vi "Remove JSON Tag.vi"(11 "Name":string) -> (2 "Tag":T1, 3 "Name (tag stripped)":string)   [LabVIEW 2024, in "JSONtext.lvlib"]
uses:
  JSONtext.lvlib
  Tag Type.ctl
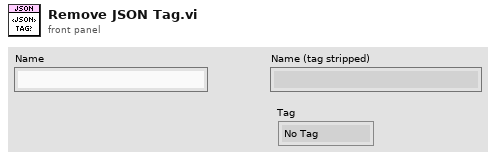
[diagram p1: front panel]
types:
  T1 = typedef "JSONtext.lvlib/Tag Type.ctl" = enum16{"No Tag", "<JSON>", "<JOBJ>", "<UTF8>"}
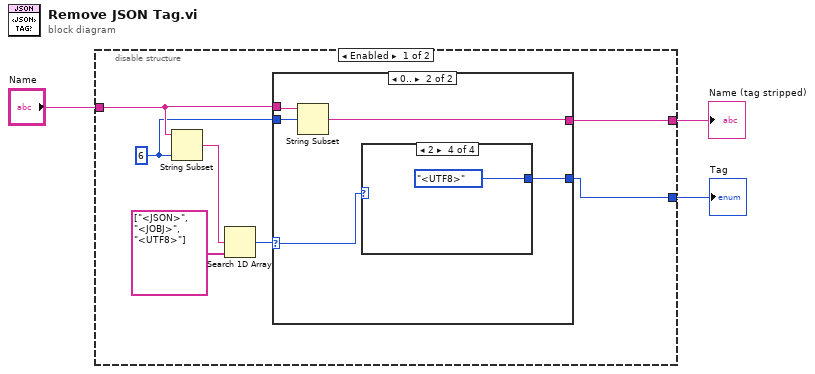
[diagram p0: block diagram]
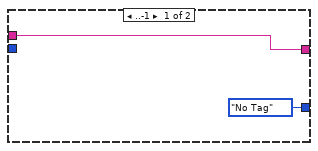
[diagram p2: hidden frame]
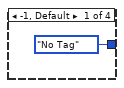
[diagram p3: hidden frame]
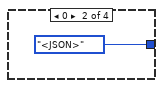
[diagram p4: hidden frame]
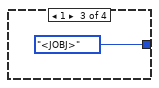
[diagram p5: hidden frame]
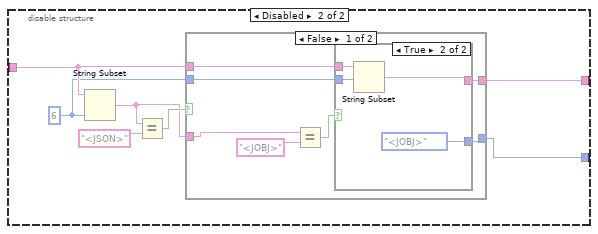
[diagram p6: hidden frame]
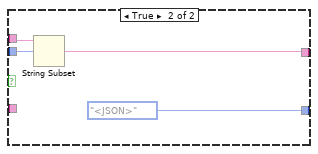
[diagram p8: hidden frame]
diagram:
  n1 = disable-structure shown="Enabled" {
    disable-tunnel: "Name" -> [w10 w27]
    disable-tunnel: [w9 w26] -> w2
    disable-tunnel: [w7 w22] -> w1
    frame Enabled {
      w8 = 6 ("length (rest)")
      n2 = String Subset(string=w10, length (rest)=w8) -> (substring=w5:string)  [unwired: 1 in]
      n3 = Search 1D Array(1D array=string[] ["<JSON>", "<JOBJ>", "<UTF8>"], element=w5) -> (index of element=w4:i32)  [unwired: 1 in]
      n4 = case shown="0.." w4 {
        selector: w4 -> [_ w14]
        tunnel: [w12 w16] -> w9
        tunnel: w10 -> [w12 w17]
        tunnel: w8 -> [_ w13]
        tunnel: [Tag_Type."No Tag" ("Tag") w15] -> w7
        frame ..-1 {
        }
        frame 0.. {
          n5 = String Subset(string=w17, offset (0)=w13) -> (substring=w16:string)  [unwired: 1 in]
          n6 = case shown="2" w14 {
            tunnel: [Tag_Type."No Tag" ("Tag") Tag_Type."<JSON>" ("Tag") Tag_Type."<JOBJ>" ("Tag") Tag_Type."<UTF8>" ("Tag")] -> w15
            frame -1, Default {
            }
            frame 0 {
            }
            frame 1 {
            }
            frame 2 {
            }
          }
        }
      }
    }
    frame Disabled {
      w24 = 6 ("length (rest)")
      n7 = String Subset(string=w27, length (rest)=w24) -> (substring=w23:string)  [unwired: 1 in]
      n8 = Equal?(x=w23, y="<JSON>") -> (x = y?=w28:bool)
      n9 = case shown="False" w28 {
        tunnel: [w32 w43] -> w26
        tunnel: w27 -> [w33 w44]
        tunnel: w24 -> [w31 w42]
        tunnel: w23 -> [w34 _]
        tunnel: [w29 Tag_Type."<JSON>" ("Tag")] -> w22
        frame False {
          n10 = Equal?(x=w34, y="<JOBJ>") -> (x = y?=w30:bool)
          n11 = case shown="True" w30 {
            tunnel: w33 -> [w36 w40]
            tunnel: [w36 w39] -> w32
            tunnel: w31 -> [_ w38]
            tunnel: [_ Tag_Type."<JOBJ>" ("Tag")] -> w29
            frame False {
            }
            frame True {
              n12 = String Subset(string=w40, offset (0)=w38) -> (substring=w39:string)  [unwired: 1 in]
            }
          }
        }
        frame True {
          n13 = String Subset(string=w44, offset (0)=w42) -> (substring=w43:string)  [unwired: 1 in]
        }
      }
    }
  }
  "Tag" <- w1
  "Name (tag stripped)" <- w2
